vi "任务添加对话框.vi"(8 "error in (no error)":errorcluster, 11 "Cleaningcycle in":refnum<class "Cleaning cycle.lvclass">) -> (0 "error out":errorcluster, 1 "项名":string[](array[string]), 2 "check?":bool, 3 "Cleaningcycle out":refnum<class "Cleaning cycle.lvclass">)   [LabVIEW 2022 SP3, in "Cleaning cycle.lvclass"]
uses:
  Cleaning cycle.lvclass
panel:
  in  "分":T1(ring)
  in  "时":T2(ring)
  in  "频次":T3(ring)
  in  "取消":bool
  in  "确定":bool
  in  "参数":u32(ring)
  in  "任务项":u32(ring)
  # "启动时间"
  # "："
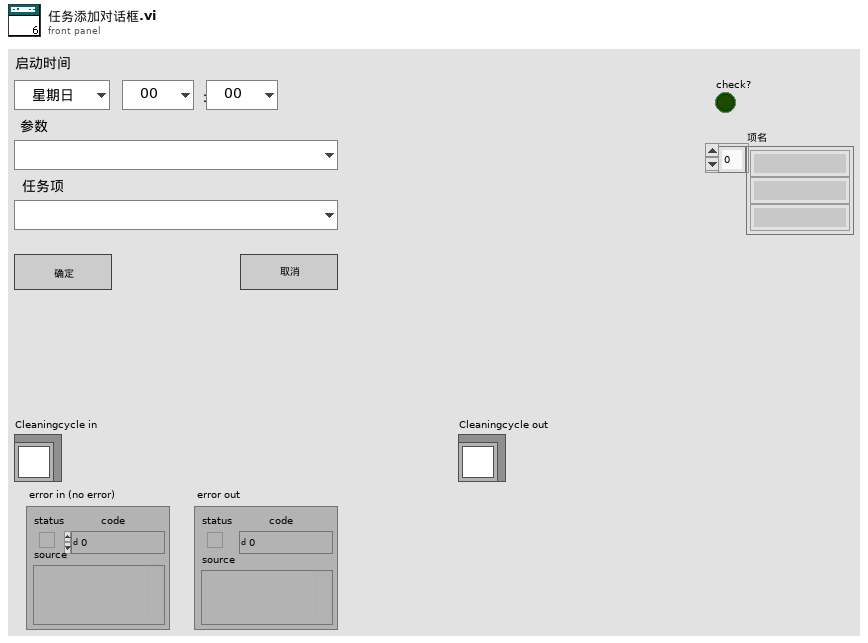
[diagram p1: front panel]
types:
  T1 = enum16{"00", "01", "02", "03", "04", "05", "06", "07", "08", "09", "10", "11", "12", "13", "14", "15", "16", "17", "18", "19", "20", "21", "22", "23", "24", "25", "26", "27", "28", "29", "30", "31", "32", "33", "34", "35", "36", "37", "38", "39", "40", "41", "42", "43", "44", "45", "46", "47", "48", "49", "50", "51", "52", "53", "54", "55", "56", "57", "58", "59"}
  T2 = enum16{"00", "01", "02", "03", "04", "05", "06", "07", "08", "09", "10", "11", "12", "13", "14", "15", "16", "17", "18", "19", "20", "21", "22", "23"}
  T3 = enum16{"星期日", "星期一", "星期二", "星期三", "星期四", "星期五", "星期六", "每天"}
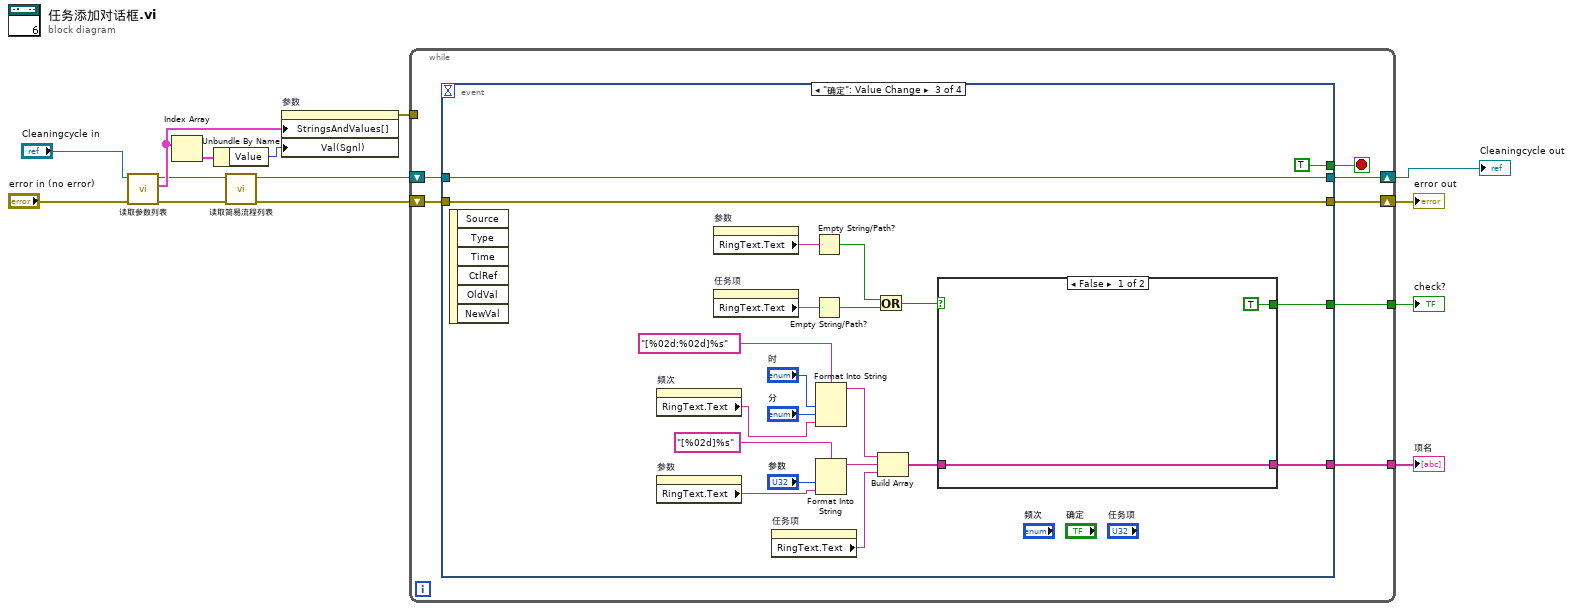
[diagram p0: block diagram]
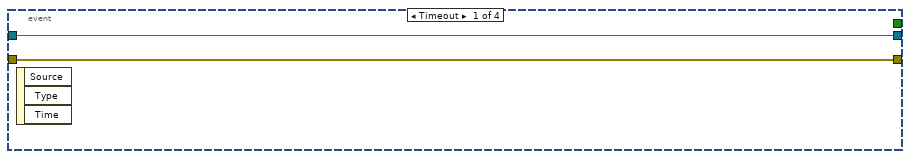
[diagram p2: hidden frame]
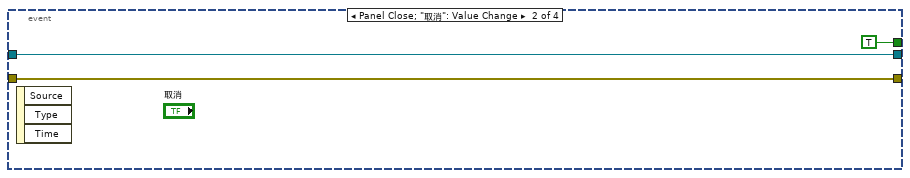
[diagram p3: hidden frame]
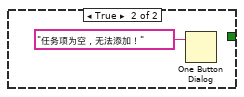
[diagram p4: hidden frame]
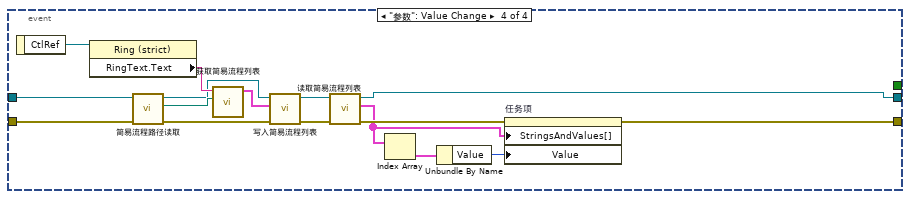
[diagram p5: hidden frame]
diagram:
  n1 = call "读取参数列表.vi"("error in (no error)"="error in (no error)", "Cleaningcycle 输入"="Cleaningcycle in") -> ("error out"=w4:errorcluster, "参数列表"=w8:cluster{"String":string, "Value":u16}[], "Cleaningcycle 输出"=w5:refnum<class "Cleaning cycle.lvclass">)  [unwired: 7 in]
  n2 = Index Array(array=w8) -> (element=w14:cluster{"String":string, "Value":u16})  [unwired: 1 in]
  n3 = Unbundle By Name(w14) -> ("Value"=w13:u16)
  n4 = call "读取简易流程列表.vi"("error in (no error)"=w4, "Cleaningcycle 输入"=w5) -> ("error out"=w2:errorcluster, "Cleaningcycle 输出"=w3:refnum<class "Cleaning cycle.lvclass">)  [unwired: 7 in, 1 out]
  n5 = property on="参数" class="Ring (strict)"("StringsAndValues[]"=w8, "Val(Sgnl)"=w13) -> (error out=w1:errorcluster)  [unwired: 2 in, 1 out]
  n6 = while {
    tunnel: [w20] -> w12
    tunnel: [w19] -> w11
    shift-right: [w16] -> w6
    shift-left: w3 -> [w18]
    shift-right: [w15] -> w7
    shift-left: w2 -> [w17]
    tunnel: w1 -> [_]
    stop <- w21 stop-if-true
    n7 = event shown="[2] \"确定\": Value Change" {
      selector: _ -> [_ _ _ _]
      dyn-events: _ -> [_ _ _ _]
      timeout: _ -> [_ _ _ _]
      tunnel: [_ TRUE TRUE _] -> w21
      tunnel: [_ _ w43 _] -> w20
      tunnel: [_ _ w41 _] -> w19
      tunnel: w18 -> [w23 w25 w40 w64]
      tunnel: w17 -> [w22 w24 w39 w63]
      tunnel: [w23 w25 w40 w51] -> w16
      tunnel: [w22 w24 w39 w54] -> w15
      event Timeout {
        n8 = event-data() -> ()  [unwired: 1 in, 3 out]
      }
      event Panel Close; "取消": Value Change {
        n9 = event-data() -> ()  [unwired: 1 in, 3 out]
      }
      event "确定": Value Change {
        n10 = event-data() -> ()  [unwired: 1 in, 6 out]
        n11 = property on="频次" class="Enum (strict)"() -> ("RingText.Text"=w27:string)  [unwired: 2 in, 2 out]
        n12 = property on="参数" class="Ring (strict)"() -> ("RingText.Text"=w30:string)  [unwired: 2 in, 2 out]
        n13 = property on="参数" class="Ring (strict)"() -> ("RingText.Text"=w37:string)  [unwired: 2 in, 2 out]
        n14 = property on="任务项" class="Ring (strict)"() -> ("RingText.Text"=w38:string)  [unwired: 2 in, 2 out]
        n15 = property on="任务项" class="Ring (strict)"() -> ("RingText.Text"=w32:string)  [unwired: 2 in, 2 out]
        n16 = Empty String/Path?(string/path=w37) -> (empty?=w45:bool)
        n17 = Empty String/Path?(string/path=w38) -> (empty?=w46:bool)
        n18 = Format Into String(format string="[%02d:%02d]%s" ("格式字符串"), "时", "分", w27) -> (resulting string=w35:string)  [unwired: 2 in, 1 out]
        n19 = Format Into String(format string="[%02d]%s" ("格式字符串"), "参数", w30) -> (resulting string=w33:string)  [unwired: 2 in, 1 out]
        n20 = Or(x=w45, y=w46) -> (x .or. y?=w44:bool)
        n21 = Build Array(w35, w33, w32) -> (w42:string[])
        n22 = case shown="False" w44 {
          tunnel: [TRUE _] -> w43
          tunnel: w42 -> [w48 _]
          tunnel: [w48 _] -> w41
          frame False {
          }
          frame True {
            n23 = One Button Dialog(message="任务项为空，无法添加！" ("消息")) -> ()  [unwired: 1 in, 1 out]
          }
        }
      }
      event "参数": Value Change {
        n24 = event-data() -> ("CtlRef"=w66:refnum<vi>)  [unwired: 1 in]
        n25 = property class="Ring (strict)"(reference=w66) -> ("RingText.Text"=w65:string)  [unwired: 1 in, 2 out]
        n26 = call "简易流程路径读取.vi"("error in (no error)"=w63, "Cleaningcycle 输入"=w64) -> ("error out"=w60:errorcluster, "简易流程路径"=w62:path, "Cleaningcycle 输出"=w61:refnum<class "Cleaning cycle.lvclass">)  [unwired: 7 in]
        n27 = call "获取简易流程列表.vi"("添加的路径"=w62, "查询参数"=w65) -> ("简易流程列表"=w59:cluster{"String":string, "Value":u16}[])  [unwired: 8 in, 1 out]
        n28 = call "写入简易流程列表.vi"("error in (no error)"=w60, "简易流程列表"=w59, "Cleaningcycle 输入"=w61) -> ("error out"=w56:errorcluster, "Cleaningcycle 输出"=w57:refnum<class "Cleaning cycle.lvclass">)  [unwired: 7 in]
        n29 = call "读取简易流程列表.vi"("error in (no error)"=w56, "Cleaningcycle 输入"=w57) -> ("error out"=w55:errorcluster, "简易流程列表"=w52:cluster{"String":string, "Value":u16}[], "Cleaningcycle 输出"=w51:refnum<class "Cleaning cycle.lvclass">)  [unwired: 7 in]
        n30 = Index Array(array=w52) -> (element=w58:cluster{"String":string, "Value":u16})  [unwired: 1 in]
        n31 = Unbundle By Name(w58) -> ("Value"=w53:u16)
        n32 = property on="任务项" class="Ring (strict)"(error in=w55, "StringsAndValues[]"=w52, "Value"=w53) -> (error out=w54:errorcluster)  [unwired: 1 in, 1 out]
      }
    }
  }
  "check?" <- w12
  "项名" <- w11
  "Cleaningcycle out" <- w6
  "error out" <- w7
